vi "FP_Apply_digital_signature.vi"(8 "Error In":errorcluster, 10 "Path to EXE to sign":path, 11 "Path to Signtool folder":path=path "C:/Program Files (x86)/Windows Kits/10/bin/10.0.19041.0/x64") -> (0 "Error Out":errorcluster, 2 "Error":string, 3 "Message":string)   [LabVIEW 2018]
uses:
  <vilib>/Utility/miscctls.llb/LVPointTypeDef.ctl
  <userlib>/_OpenG.lib/file/file.llb/Valid Path - Traditional__ogtk.vi
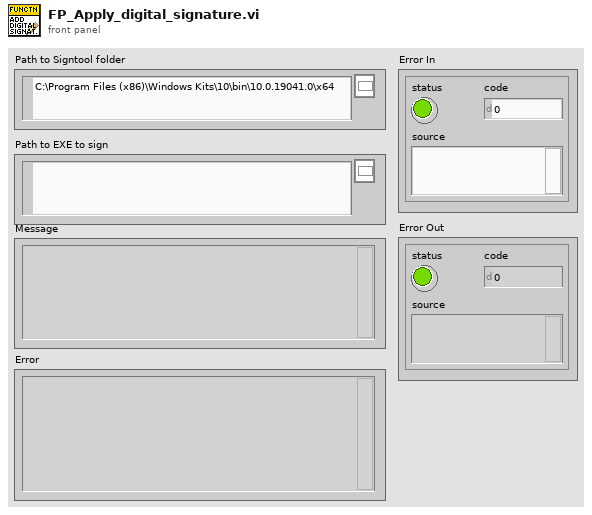
[diagram p1: front panel]
types:
  T1 = typedef "LVPointTypeDef.ctl" = cluster{"Horizontal":i16, "Vertical":i16}
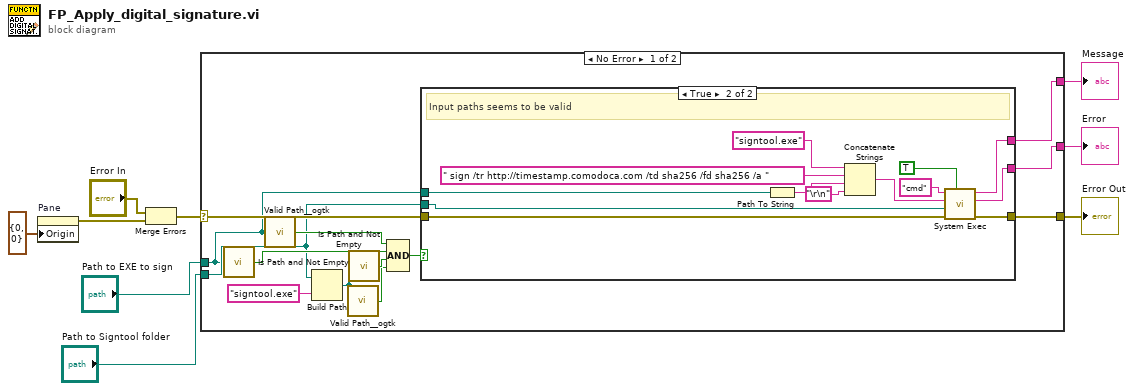
[diagram p0: block diagram]
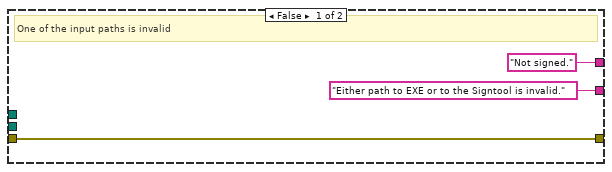
[diagram p2: hidden frame]
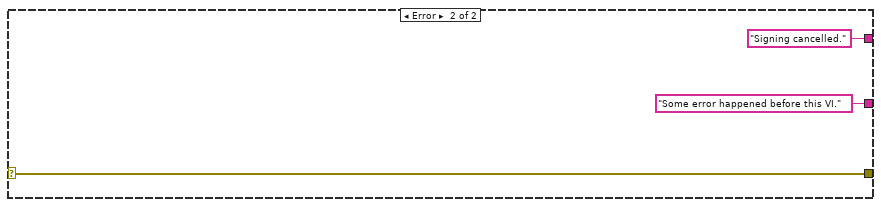
[diagram p3: hidden frame]
diagram:
  n1 = property on="Pane" class="Pane"("Origin"=T1 {"Horizontal"=0, "Vertical"=0}) -> (error out=w1:errorcluster)  [unwired: 2 in, 1 out]
  n2 = Merge Errors("Error In", w1) -> (w2:errorcluster)
  n3 = case shown="No Error" w2 {
    selector: w2 -> [w14 w41]
    tunnel: [w15 w41] -> w8
    tunnel: [w13 "Signing cancelled." ("standard output")] -> w7
    tunnel: "Path to Signtool folder" -> [w12 _]
    tunnel: "Path to EXE to sign" -> [w11 _]
    tunnel: [w10 "Some error happened before this VI."] -> w4
    frame No Error {
      n4 = call <vilib>:"Is Path and Not Empty.vi"("path"=w11) -> ("Is Path and Not Empty?"=w19:bool)  [unwired: 4 in]
      n5 = call-poly <userlib>:"Valid Path__ogtk.vi"("path"=w11) -> ("valid"=w20:bool)
      n6 = Build Path(base path=w12, name or relative path="signtool.exe") -> (appended path=w22:path)
      n7 = call-poly <userlib>:"Valid Path__ogtk.vi"("path"=w22) -> ("valid"=w17:bool)
      n8 = call <vilib>:"Is Path and Not Empty.vi"("path"=w22) -> ("Is Path and Not Empty?"=w18:bool)  [unwired: 4 in]
      n9 = Compound Arithmetic op=AND(w20, w19, w18, w17) -> (w16:bool)
      n10 = case shown="True" w16 {
        tunnel: [w25 w35] -> w15
        tunnel: w14 -> [w25 w36]
        tunnel: ["Not signed." ("standard output") w27] -> w13
        tunnel: w12 -> [_ w37]
        tunnel: w11 -> [_ w29]
        tunnel: ["Either path to EXE or to the Signtool is invalid." w26] -> w10
        frame False {
          # "One of the input paths is invalid"
        }
        frame True {
          # "Input paths seems to be valid"
          n11 = Path To String(path=w29) -> (string=w31:string)
          n12 = Concatenate Strings("signtool.exe" ("string"), " sign /tr http://timestamp.comodoca.com /td sha256 /fd sha256 /a " ("string"), w31, "\r\n") -> (w33:string)
          n13 = call <vilib>:"System Exec.vi"("wait until completion? (T)"=TRUE, "error in (no error)"=w36, "working directory"=w37, "standard input"=w33, "command line"="cmd") -> ("error out"=w35:errorcluster, "standard error"=w26:string, "standard output"=w27:string)  [unwired: 3 in, 1 out]
        }
      }
    }
    frame Error {
    }
  }
  "Error Out" <- w8
  "Message" <- w7
  "Error" <- w4
